vi "Configure Modulation(Amplitude).vi"(0 "VISA resource name":refnum<visa-resource-name>, 1 "Enable Amplitude Modulation (F: Disable)":bool, 2 "Modulation Depth (100 %)":dbl=100.0, 5 "Channel (1: Channel 1)":i32(ring)=1 items=["Channel 1"=1, "Channel 2"=2], 7 "AM Source (0: Internal)":i32(ring) items=["Internal", "External"], 9 "Modulation Waveform (0: Sinusoid)":i32(ring) items=["Sinusoid", "Square", "Triangle", "Ramp", "Nramp", "Noise", "User"], 11 "error in (no error)":errorcluster, 12 "Modulation Frequency (100 Hz)":dbl=100.0) -> (4 "VISA resource name out":refnum<visa-resource-name>, 15 "error out":errorcluster)   [LabVIEW 2012, in "RIGOL DG4000 Series.lvlib"]
doc: "Configures amplitude modulation."
uses:
  <instrlib>/RIGOL DG4000 Series/RIGOL DG4000 Series.lvlib
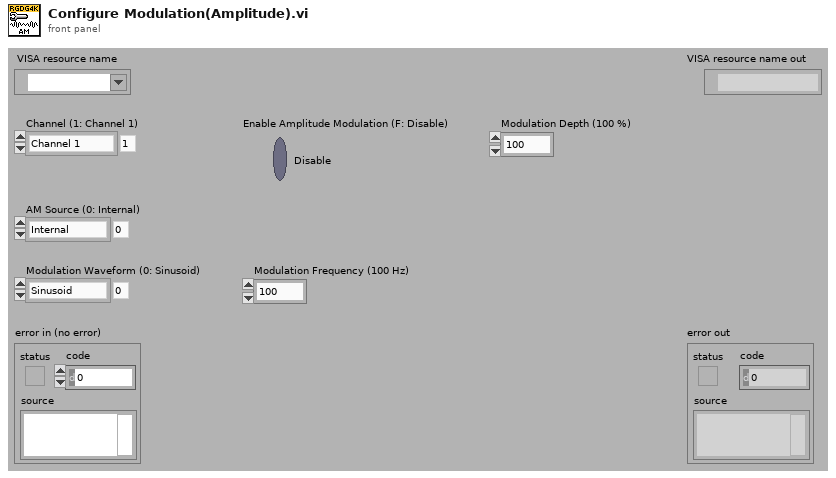
[diagram p1: front panel]
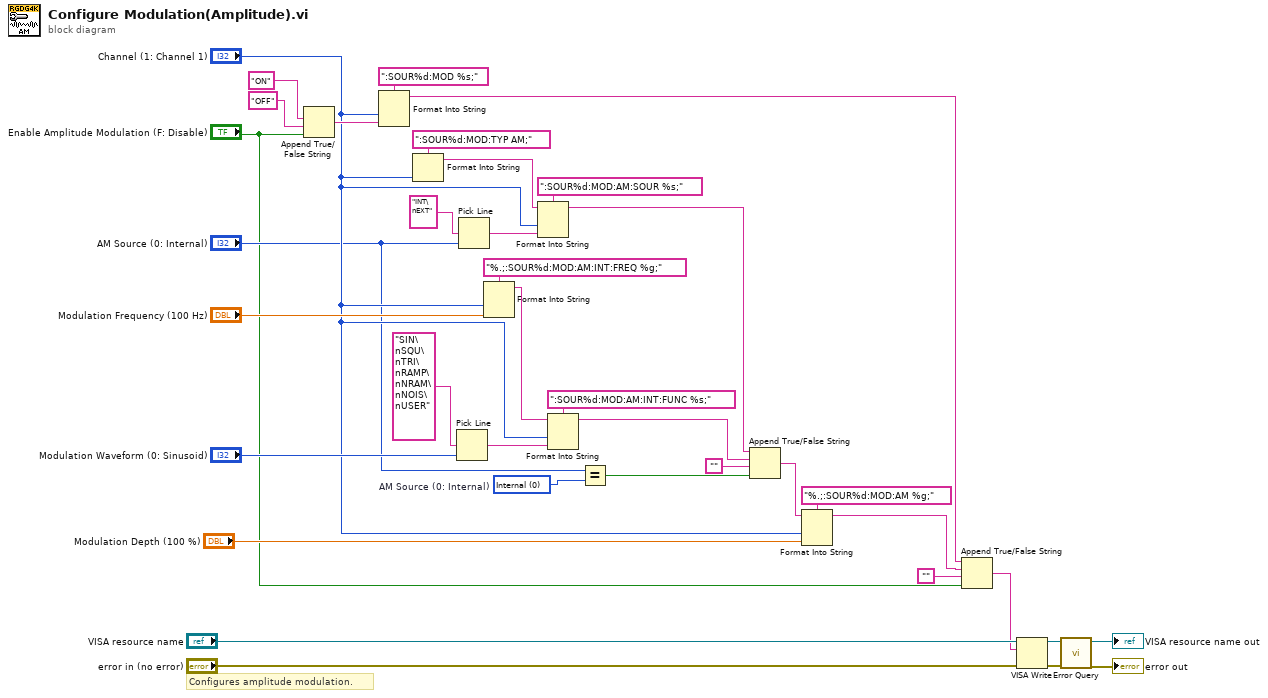
[diagram p0: block diagram]
diagram:
  w8 = 0 items=["Internal", "External"]  # AM Source (0: Internal)
  # "Configures amplitude modulation."
  n1 = Append True/False String(1:"Enable Amplitude Modulation (F: Disable)", 2:"OFF", 3:"ON") -> (0:w34:string)  [unwired: 1 out]
  n2 = Format Into String(format string=":SOUR%d:MOD %s;", "Channel (1: Channel 1)", w34) -> (resulting string=w4:string)  [unwired: 2 in, 1 out]
  n3 = Format Into String(format string=":SOUR%d:MOD:TYP AM;", "Channel (1: Channel 1)") -> (resulting string=w15:string)  [unwired: 2 in, 1 out]
  n4 = Pick Line(multi-line string="SIN\nSQU\nTRI\nRAMP\nNRAM\nNOIS\nUSER", line index="Modulation Waveform (0: Sinusoid)") -> (output string=w25:string)  [unwired: 1 out]
  n5 = Pick Line(multi-line string="INT\nEXT", line index="AM Source (0: Internal)") -> (output string=w22:string)  [unwired: 1 out]
  n6 = Format Into String(format string="%.;:SOUR%d:MOD:AM:INT:FREQ %g;", "Channel (1: Channel 1)", "Modulation Frequency (100 Hz)") -> (resulting string=w27:string)  [unwired: 2 in, 1 out]
  n7 = Format Into String(format string=":SOUR%d:MOD:AM:SOUR %s;", initial string=w15, "Channel (1: Channel 1)", w22) -> (resulting string=w12:string)  [unwired: 1 in, 1 out]
  n8 = Format Into String(format string=":SOUR%d:MOD:AM:INT:FUNC %s;", initial string=w27, "Channel (1: Channel 1)", w25) -> (resulting string=w13:string)  [unwired: 1 in, 1 out]
  n9 = Equal?(x="AM Source (0: Internal)", y=w8) -> (x = y?=w6:bool)
  n10 = Append True/False String(1:w6, 2:"", 3:w13, 4:w12) -> (0:w9:string)
  n11 = Format Into String(format string="%.;:SOUR%d:MOD:AM %g;", initial string=w9, "Channel (1: Channel 1)", "Modulation Depth (100 %)") -> (resulting string=w3:string)  [unwired: 1 in, 1 out]
  n12 = Append True/False String(1:"Enable Amplitude Modulation (F: Disable)", 2:"", 3:w3, 4:w4) -> (0:w1:string)
  n13 = VISA Write(VISA resource name="VISA resource name", write buffer=w1, error in (no error)="error in (no error)") -> (VISA resource name out=w19:refnum<visa-resource-name>, error out=w18:errorcluster)  [unwired: 1 out]
  n14 = call <instrlib>:"Error Query.vi"("error in (no error)"=w18, "VISA resource name"=w19) -> ("error out"=→"error out":errorcluster, "VISA resource name out"=→"VISA resource name out":refnum<visa-resource-name>)  [unwired: 8 out]
